vi "InitHardware.vi"(8 "error in (no error)":errorcluster, 11 "Point Grey Camera in":refnum<class "Point Grey Camera.lvclass">) -> (0 "error out":errorcluster, 1 "bit depth":string, 2 "Image Type":T1 items=["Grayscale (U8)", "Grayscale (I16)", "Grayscale (SGL)", "Complex (CSG)", "RGB (U32)", "HSL (U32)", "RGB (U64)", "Grayscale (U16)"], 3 "Point Grey Camera out":refnum<class "Point Grey Camera.lvclass">)   [LabVIEW 2020, in "Point Grey Camera.lvclass"]
uses:
  Point Grey Camera.lvclass
  Point Grey Camera.lvclass/Point Grey Camera.ctl
  NI_Vision_Acquisition_Software.lvlib
  C:/Program Files (x86)/National Instruments/LabVIEW 2020/resource/objmgr/imaqdx.rc
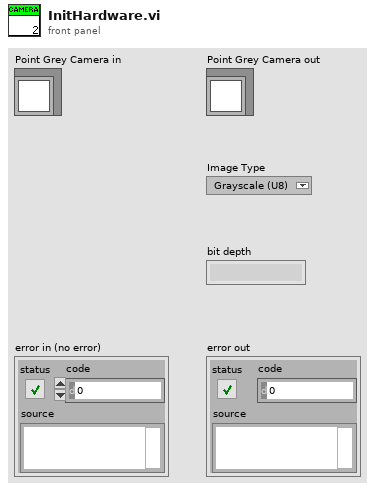
[diagram p1: front panel]
types:
  T1 = typedef "Image Type" = u32
  T2 = typedef "OnOffTypeDef.ctl" = enum16{"off", "on"}
  T3 = typedef "TriggerModeString_TypDEf.ctl" = cluster{"On":string, "Off":string}
  T4 = typedef "CamAtributes_TypDEf.ctl" = cluster{"Gain":string, "Shutter":string, "TriggerDelay":string, "TriggerMode":string, "ROI Width":string, "ROI Height":string, "ROI OffsetX":string, "ROI OffsetY":string}
  T5 = typedef "IMAQdx.ctl" = refnum<k21>
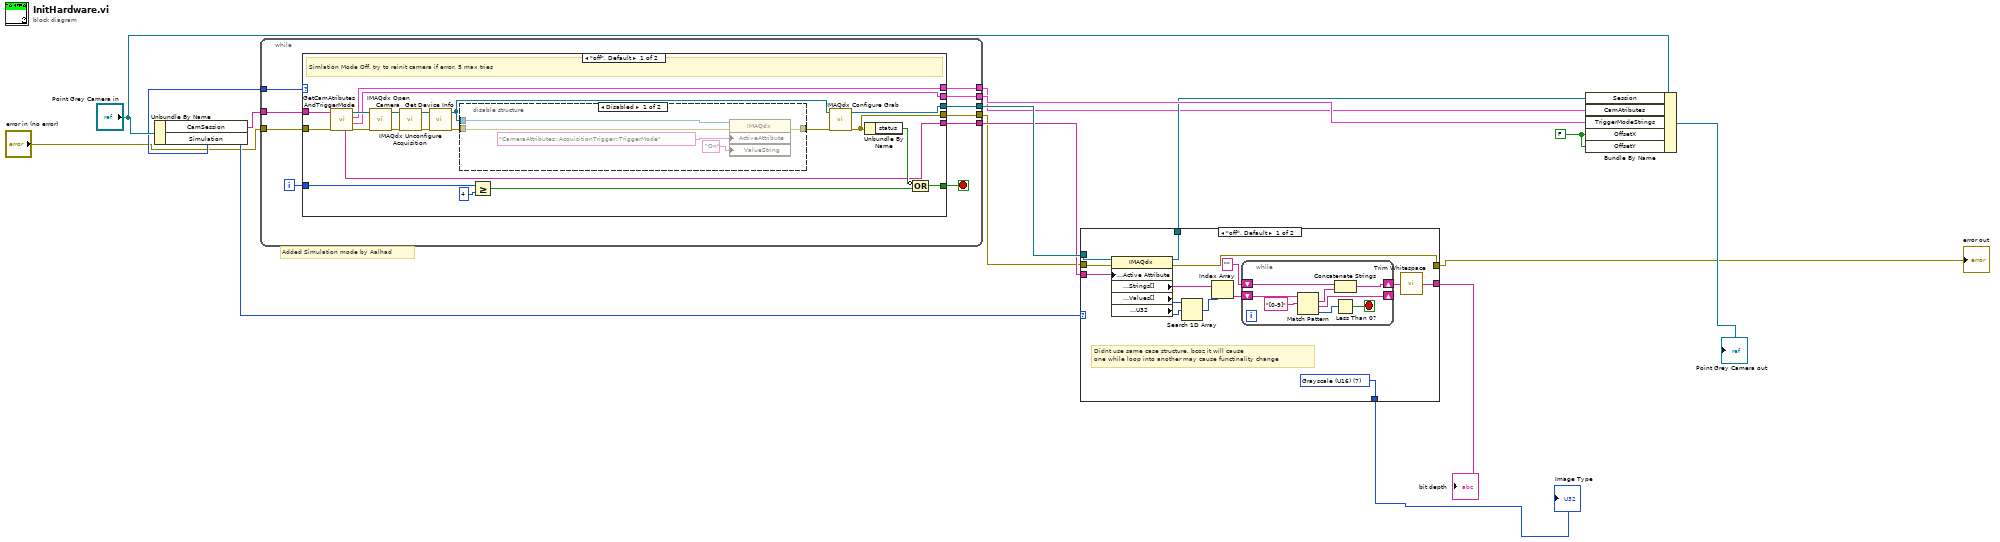
[diagram p0: block diagram]
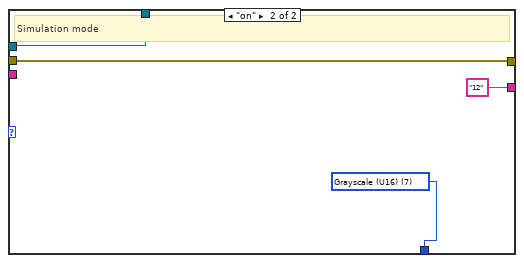
[diagram p2: hidden frame]
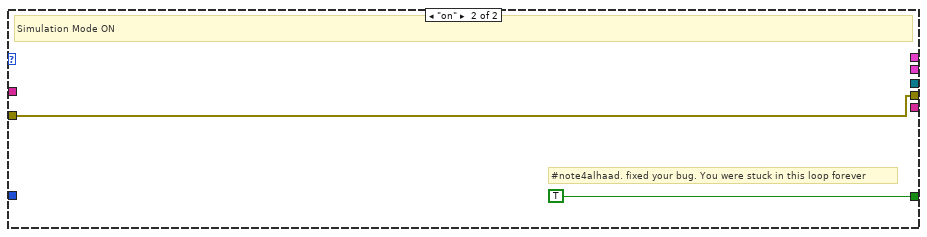
[diagram p4: hidden frame]
diagram:
  w3 = FALSE ("OffsetX")
  # "Added Simulation mode by Aalhad"
  n1 = Unbundle By Name("Point Grey Camera in") -> ("CamSession"=w2:string, "Simulation"=w9:T2)
  n2 = while "try to reinit camera if error. 5 max tries" {
    tunnel: [w25] -> w1
    tunnel: [w24] -> w10
    tunnel: "error in (no error)" -> [w23]
    tunnel: w2 -> [w22]
    tunnel: [w20] -> w4
    tunnel: [w18] -> w8
    tunnel: w9 -> [w17]
    tunnel: [w16] -> w11
    i -> [w21]
    stop <- w19 stop-if-true
    n3 = case shown="\"off\", Default" w17 {
      tunnel: [w46 _] -> w16
      tunnel: [w43 _] -> w25
      tunnel: [w42 _] -> w24
      tunnel: w23 -> [w41 w54]
      tunnel: w22 -> [w39 _]
      tunnel: w21 -> [w37 _]
      tunnel: [w35 w54] -> w20
      tunnel: [w32 TRUE] -> w19
      tunnel: [w31 _] -> w18
      frame "off", Default {
        # "Simlation Mode Off, try to reinit camera if error. 5 max tries"
        n4 = call "GetCamAtributesAndTriggerMode.vi"("error in"=w41, "IMAQdx Session"=w39) -> ("error out"=w40:errorcluster, "TriggerModeStrings"=w42:T3, "CamAtributes"=w43:T4, "IMAQdx Session 2"=w44:T5, "PixelFormat"=w31:string)  [unwired: 5 in]
        n5 = call "IMAQdx Open Camera.vi"("error in"=w40, "Session In"=w44) -> ("error out"=w45:errorcluster, "Session Out"=w38:T5)  [unwired: 1 in, 7 out]
        n6 = call "IMAQdx Unconfigure Acquisition.vi"("error in"=w45, "Session In"=w38) -> ("error out"=w28:errorcluster, "Session Out"=w29:T5)  [unwired: 8 out]
        n7 = call "Get Device Info.vi"("error in (no error)"=w28, "image in"=w29) -> ("error out"=w26:errorcluster, "image out"=w27:T5)  [unwired: 8 in]
        n8 = disable-structure shown="Disabled" {
          disable-tunnel: w27 -> [w49 _]
          disable-tunnel: w26 -> [w48 w52]
          disable-tunnel: [w47 w52] -> w30
          frame Disabled {
            n9 = property class="IMAQdx"(reference=w49, error in=w48, "ActiveAttribute"="CameraAttributes::AcquisitionTrigger::TriggerMode", "ValueString"="On") -> (error out=w47:errorcluster)  [unwired: 1 out]
          }
          frame Enabled {
          }
        }
        n10 = Greater Or Equal?(x=w37, y=4) -> (x >= y?=w33:bool)
        n11 = call "IMAQdx Configure Grab.vi"("error in"=w30, "Session In"=w27) -> ("error out"=w35:errorcluster, "Session Out"=w46:T5)  [unwired: 1 in, 7 out]
        n12 = Unbundle By Name(w35) -> ("status"=w34:bool)
        n13 = Compound Arithmetic op=OR(invert w34, w33) -> (w32:bool)
      }
      frame "on" {
        # "#note4alhaad. fixed your bug. You were stuck in this loop forever"
        # "Simulation Mode ON"
      }
    }
  }
  n14 = case shown="\"off\", Default" w9 {
    tunnel: w4 -> [w61 w78]
    tunnel: [w60 w79] -> w5
    tunnel: [w59 w78] -> w12
    tunnel: [w58 "12" ("trimmed string")] -> w7
    tunnel: w8 -> [w57 _]
    tunnel: w11 -> [w56 w79]
    tunnel: [w55 w77] -> w13
    frame "off", Default {
      w55 = T1 7 items=["Grayscale (U8)", "Grayscale (I16)", "Grayscale (SGL)", "Complex (CSG)", "RGB (U32)", "HSL (U32)", "RGB (U64)", "Grayscale (U16)"] ("Image Type")
      # "Didnt use same case structure, bcoz it will cause \none while loop into another may cause functinality change"
      n15 = property class="IMAQdx"(reference=w56, error in=w61, "Camera Attributes:Active Attribute"=w57) -> (reference out=w60:T5, error out=w59:errorcluster, "Camera Attributes:Enum:Strings[]"=w64:string[], "Camera Attributes:Enum:Values[]"=w62:u32[], "Camera Attributes:Value:U32"=w63:u32)
      n16 = Search 1D Array(1D array=w62, element=w63) -> (index of element=w65:i32)  [unwired: 1 in]
      n17 = Index Array(array=w64, index=w65) -> (element=w66:string)
      n18 = while {
        shift-right: [w74] -> _
        shift-left: w66 -> [w76]
        shift-right: [w70] -> w68
        shift-left: "" -> [w71]
        stop <- w72 stop-if-true
        n19 = Match Pattern(string=w76, regular expression="[0-9]") -> (match substring=w69:string, after substring=w74:string, offset past match=w73:i32)  [unwired: 1 in, 1 out]
        n20 = Less Than 0?(x=w73) -> (x < 0?=w72:bool)
        n21 = Concatenate Strings(w71, w69) -> (w70:string)
      }
      n22 = call "Trim Whitespace.vi"("string"=w68) -> ("trimmed string"=w58:string)  [unwired: 1 in]
    }
    frame "on" {
      w77 = T1 7 items=["Grayscale (U8)", "Grayscale (I16)", "Grayscale (SGL)", "Complex (CSG)", "RGB (U32)", "HSL (U32)", "RGB (U64)", "Grayscale (U16)"] ("Image Type")
      # "Simulation mode"
    }
  }
  "Image Type" <- w13
  "error out" <- w12
  "bit depth" <- w7
  n23 = Bundle By Name(cluster="Point Grey Camera in", "Session"=w5, "CamAtributes"=w1, "TriggerModeStrings"=w10, "OffsetX"=w3, "OffsetY"=w3) -> (→"Point Grey Camera out":refnum<class "Point Grey Camera.lvclass">)
